vi "Set Loop Period.vi"() -> ()   [LabVIEW 2019]
panel:
  in  "stop":bool
  out "Waveform Chart":dbl(graph)=-0.15643446504023392
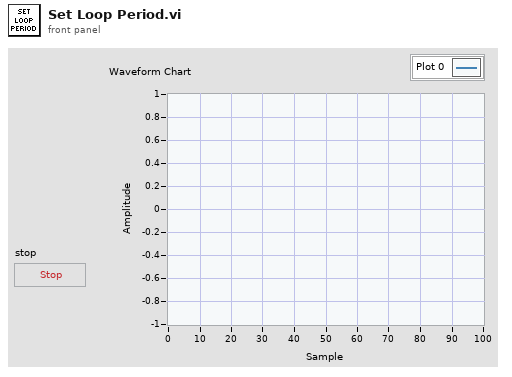
[diagram p1: front panel]
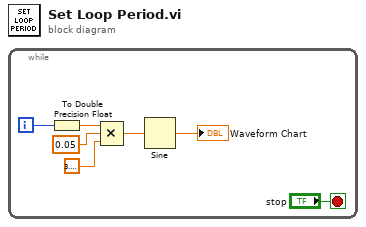
[diagram p0: block diagram]
diagram:
  n1 = while {
    i -> [w7]
    stop <- "stop" stop-if-true
    n2 = To Double Precision Float(number=w7) -> (double precision float=w6:dbl)
    n3 = Compound Arithmetic op=MULTIPLY(w6, 0.05, 3.141592653589793) -> (w3:dbl)
    n4 = Sine(x=w3) -> (sin(x)=→"Waveform Chart":dbl)
  }
